vi "REST API Test.vi"() -> ()   [LabVIEW 2017]
uses:
  <vilib>/addons/_JKI.lib/REST Client/classes/REST Client/REST Client.lvclass
  Bridge Configuration.ctl
  Result Configuration.ctl
panel:
  out "Console":string
  in  "Exit":bool
  out "Vout, V":dbl=110.0 step=100.0
  in  "Post":bool
  in  "Get":bool
  in  "R4, Ohm":dbl min=0.0 step=100.0
  in  "R3, Ohm":dbl min=0.0 step=100.0
  in  "R2, Ohm":dbl min=0.0 step=100.0
  in  "R1, Ohm":dbl min=0.0 step=100.0
  in  "Vin, V":dbl step=100.0
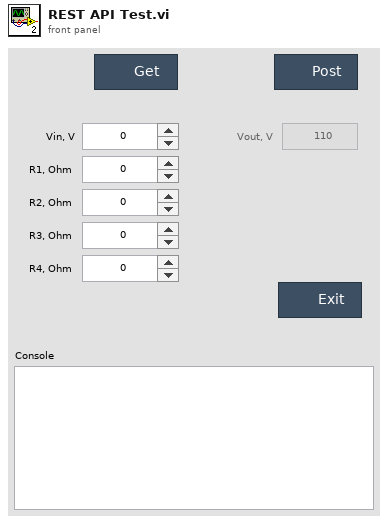
[diagram p1: front panel]
types:
  T1 = enum32{"Invalid", "Standard", "Closed", "Hidden", "Minimized", "Maximized"}
  T2 = enum32{"invalid app kind", "Development System", "Run Time System", "Student Edition", "Embedded LabVIEW", "Evaluation", "Custom"}
  T3 = typedef "Bridge Configuration.ctl" = cluster{"Vin":dbl, "R1":dbl, "R2":dbl, "R3":dbl, "R4":dbl}
  T4 = typedef "Result Configuration.ctl" = cluster{"Vout":dbl}
  T5 = cluster{"Core":cluster{"Current VI Reference":refnum<vi>, "Close Panel on Exit?":bool}, "REST Client":refnum<class "REST Client.lvclass">, "Bridge Configuration":T3, "Vout":dbl}
  T6 = cluster{"Current VI Reference":refnum<vi>, "Close Panel on Exit?":bool}
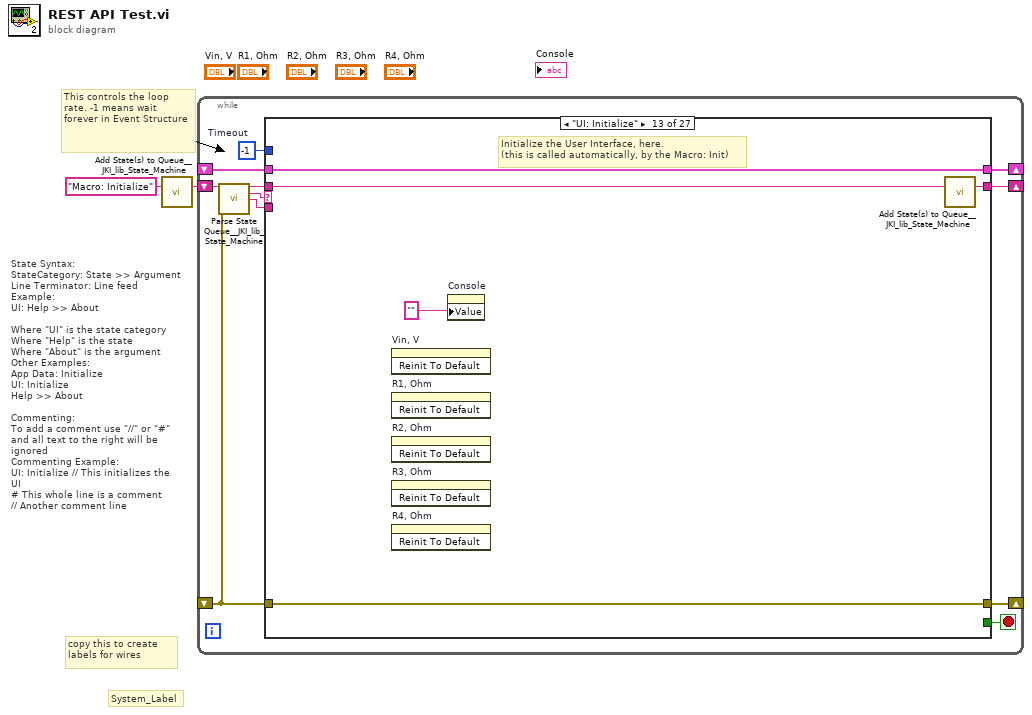
[diagram p0: block diagram]
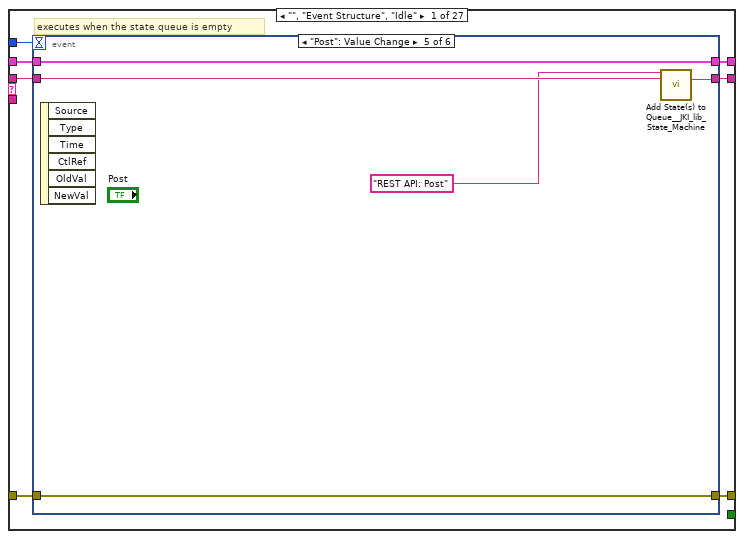
[diagram p2: hidden frame]
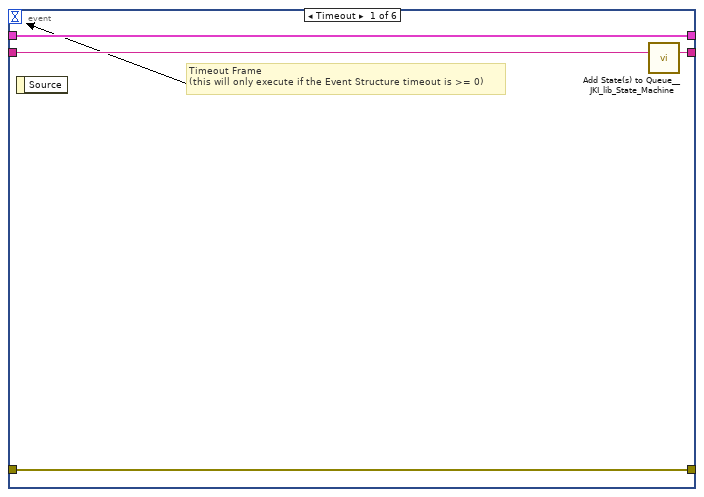
[diagram p3: hidden frame]
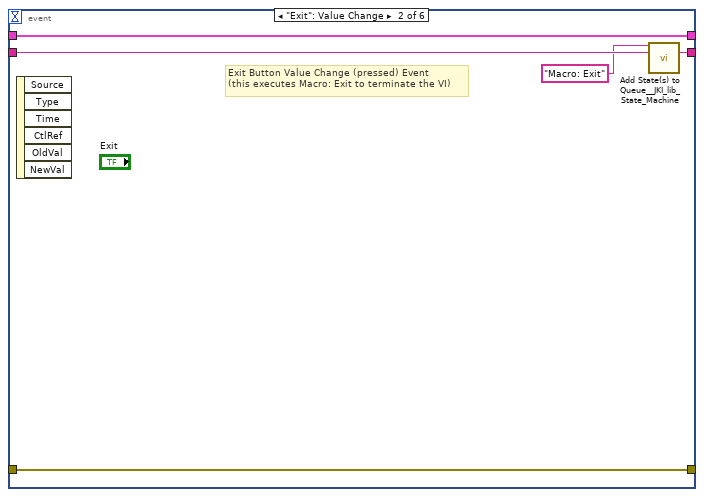
[diagram p4: hidden frame]
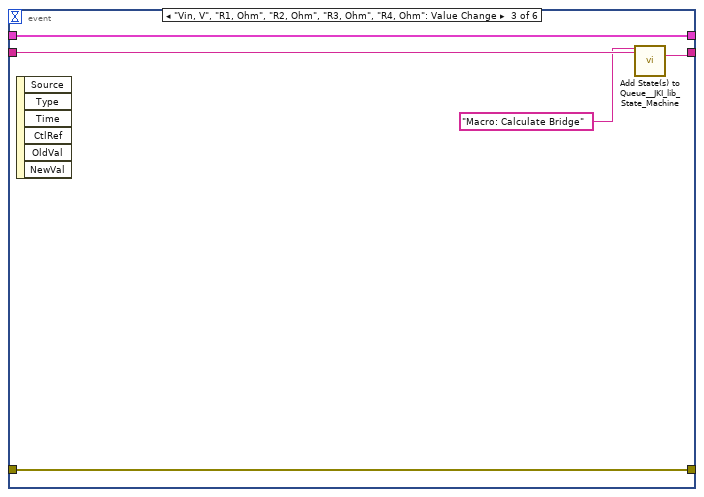
[diagram p5: hidden frame]
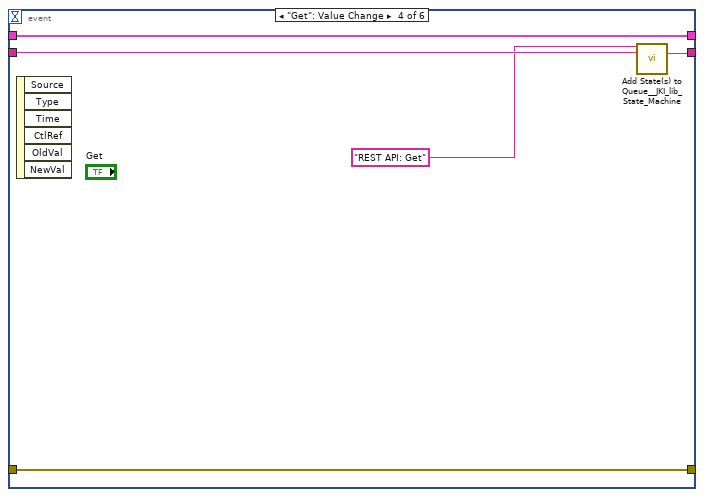
[diagram p6: hidden frame]
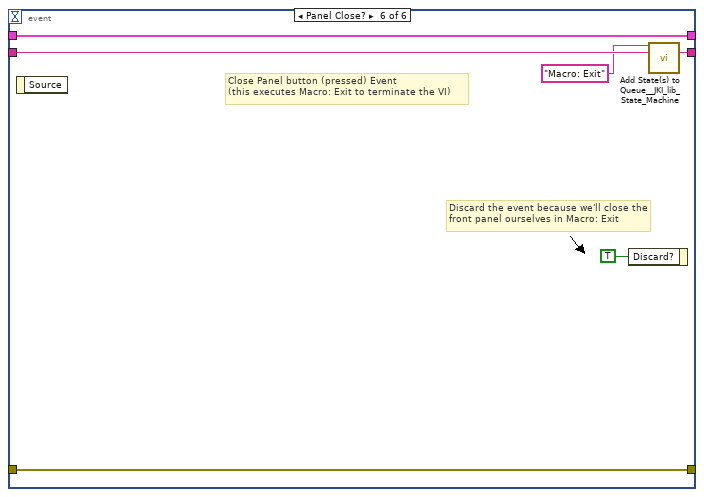
[diagram p7: hidden frame]
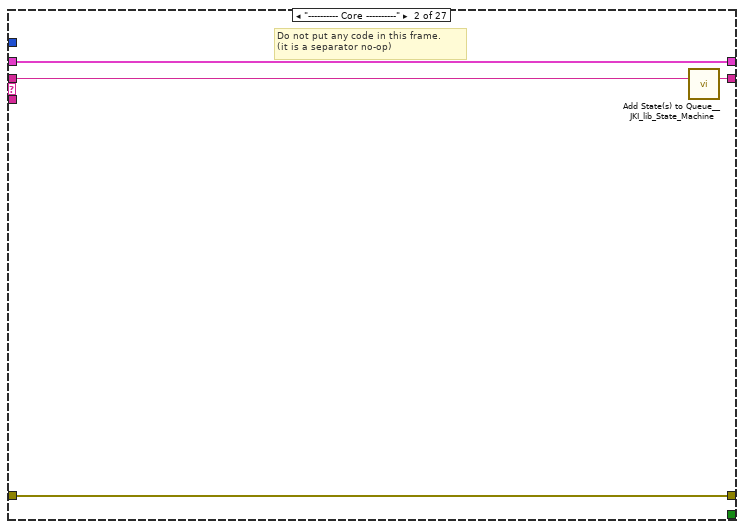
[diagram p8: hidden frame]
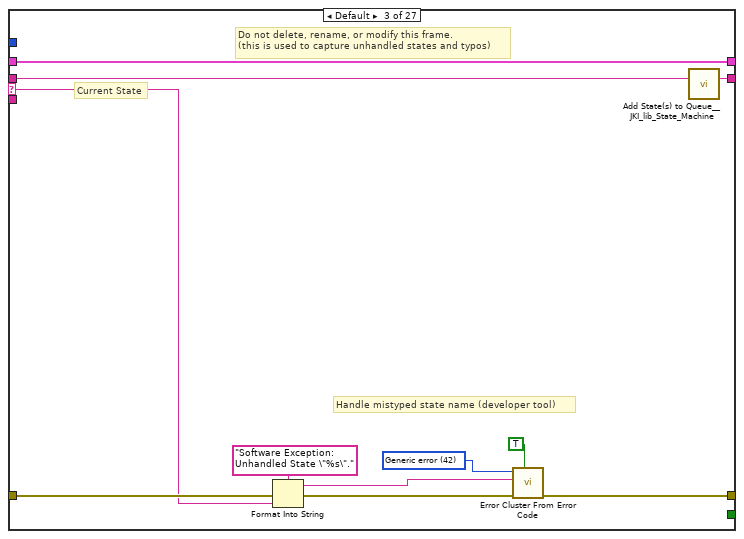
[diagram p9: hidden frame]
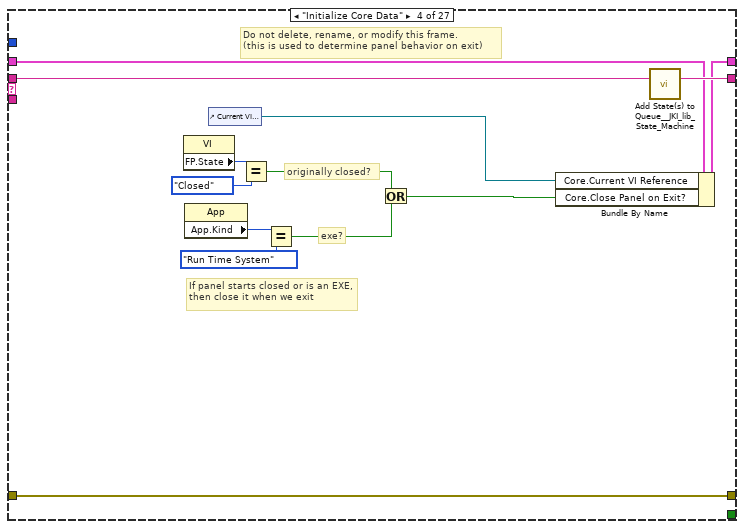
[diagram p10: hidden frame]
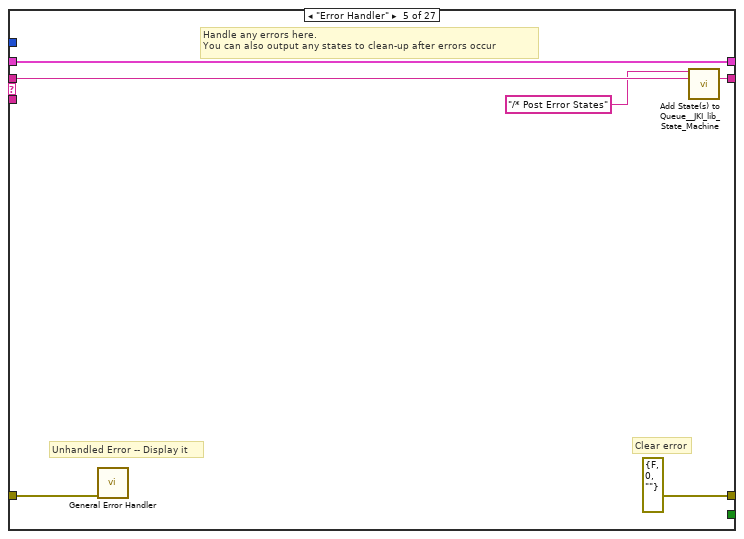
[diagram p11: hidden frame]
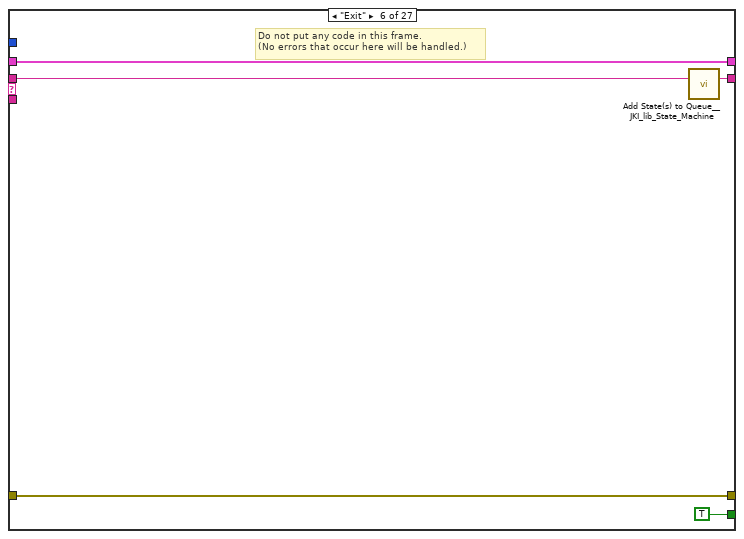
[diagram p12: hidden frame]
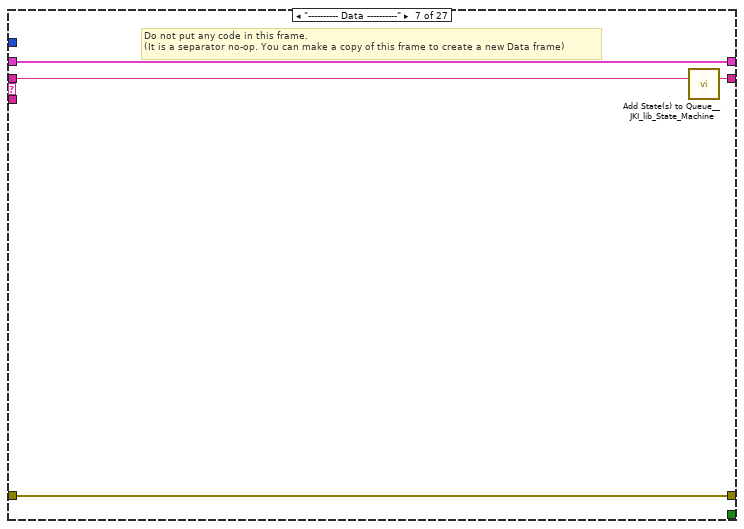
[diagram p13: hidden frame]
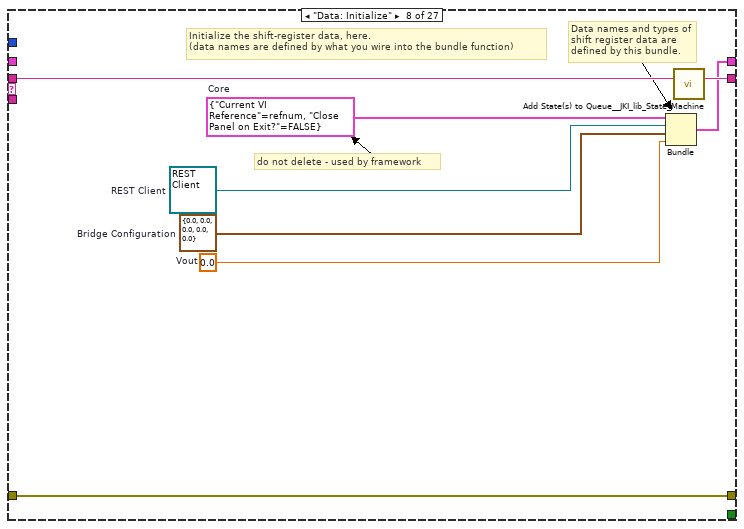
[diagram p14: hidden frame]
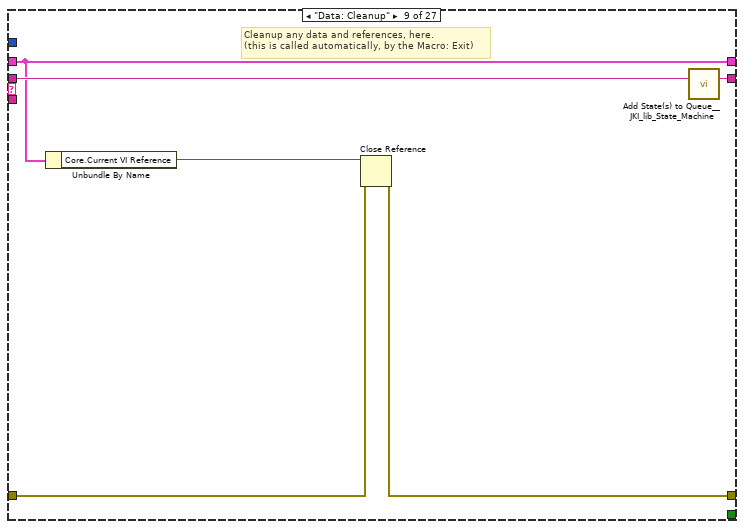
[diagram p15: hidden frame]
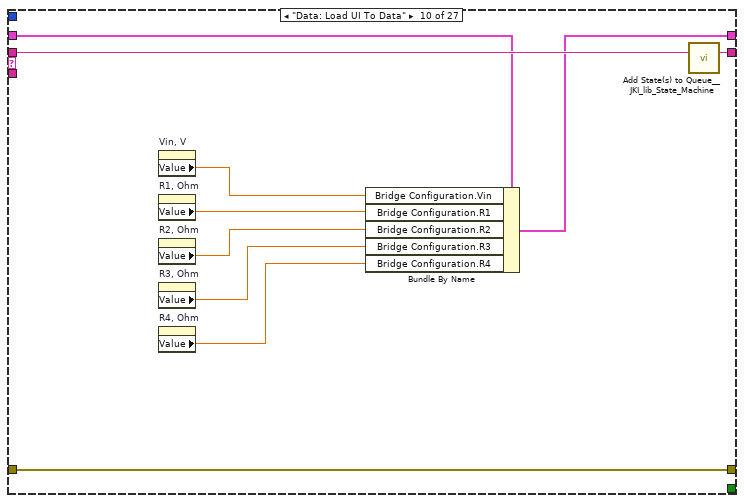
[diagram p16: hidden frame]
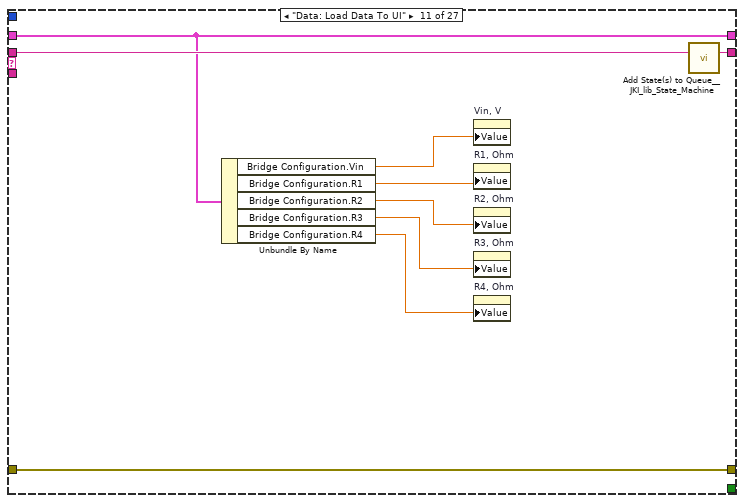
[diagram p17: hidden frame]
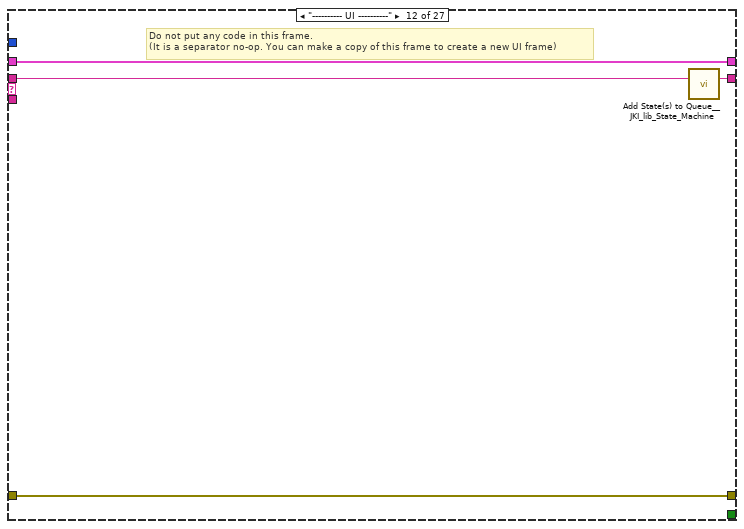
[diagram p18: hidden frame]
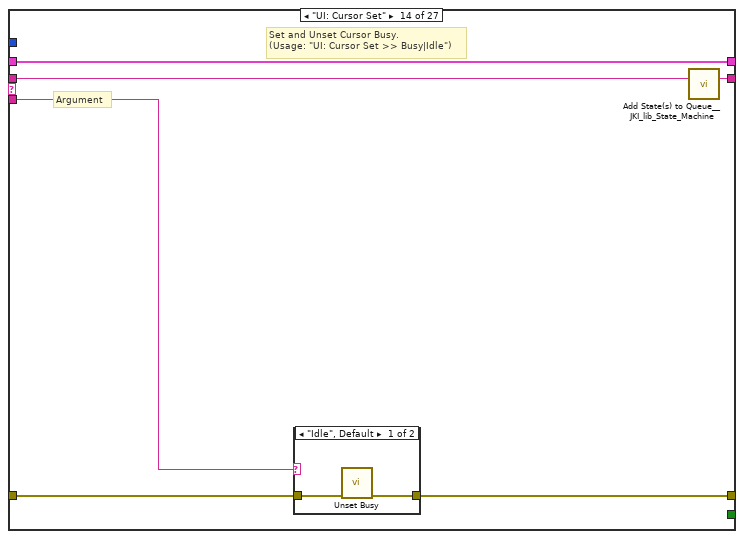
[diagram p19: hidden frame]
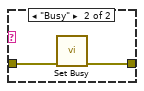
[diagram p20: hidden frame]
diagram:
  # "State Syntax:\nStateCategory: State >> Argument\nLine Terminator: Line feed\nExample:\nUI: Help >> About\n\nWhere \"UI\" is the state category\nWhere \"Help\" is the state\nWhere \"About\" is the argument\nOther Examples:\nApp Data: Initialize\nUI: Initialize\nHelp >> About\n\nCommenting:\nTo add a comment use \"//\" or \"#\" and all text to the right will be ignored\nCommenting Example:\nUI: Initialize // This initializes the UI\n# This whole line is a comment\n// Another comment line"
  # "copy this to create labels for wires"
  # "This controls the loop rate. -1 means wait forever in Event Structure"
  # "System_Label"
  n1 = call <vilib>:"Add State(s) to Queue__JKI_lib_State_Machine.vi"("State(s) in (\"\")"="Macro: Initialize") -> ("States Out"=w2:string)  [unwired: 14 in]
  n2 = while {
    shift-right: [w6] -> _
    shift-left: _ -> [w5]
    shift-right: [w9] -> _
    shift-left: _ -> [w3]
    shift-right: [w8] -> _
    shift-left: w2 -> [w10]
    stop <- w7 stop-if-true
    w4 = -1  # Timeout
    n3 = call <vilib>:"Parse State Queue__JKI_lib_State_Machine.vi"("State Queue"=w10, "Error In (no error)"=w3) -> ("Remaining States"=w12:string, "Current State"=w13:string, "Arguments"=w11:string)  [unwired: 11 in]
    n4 = case shown="\"UI: Initialize\"" w13 {
      selector: w13 -> [_ _ w55 _ _ _ _ _ _ _ _ _ _ _ _ _ _ _ _ _ _ _ _ _ _ _ _]
      tunnel: w12 -> [w20 w54 w59 w78 w84 w89 w93 w101 w107 w117 w126 w130 w135 w141 w152 w222 w226 w232 w237 w247 w251 w259 w272 w285 w291 w295 w306]
      tunnel: w11 -> [_ _ _ _ _ _ _ _ _ _ _ _ _ w136 w146 _ _ _ _ _ _ _ _ _ _ _ _]
      tunnel: w5 -> [w18 w51 w57 w71 w81 w87 w90 _ w102 w109 w118 w127 w133 w139 w148 w219 w223 w229 w234 w244 w248 w257 w264 w283 w289 w292 w298]
      tunnel: [w17 w52 w61 w75 errorcluster {"status"=FALSE, "code"=0, "source"=""} ("error out") w86 w91 w98 w103 w115 w124 w128 w132 w137 w149 w220 w224 w230 w235 w245 w249 w252 w265 w273 w286 w293 w304] -> w9
      tunnel: w3 -> [w16 w52 w60 w75 w80 w86 w91 w98 w104 w115 w124 w128 w132 w138 w150 w220 w224 w230 w235 w245 w249 w253 w267 w278 w287 w293 w304]
      tunnel: [w19 w53 w58 w77 w83 w88 w92 w100 w106 w116 w125 w129 w134 w140 w151 w221 w225 w231 w236 w246 w250 w258 w271 w284 w290 w294 w305] -> w8
      tunnel: [_ _ _ _ _ TRUE _ _ _ _ _ _ _ _ _ _ _ _ _ _ _ _ _ _ _ _ _] -> w7
      tunnel: [w15 w51 w57 w76 w81 w87 w90 w99 w102 w108 w118 w127 w133 w139 w148 w219 w223 w229 w234 w244 w248 w256 w262 w283 w289 w292 w296] -> w6
      tunnel: w4 -> [w14 _ _ _ _ _ _ _ _ _ _ _ _ _ _ _ _ _ _ _ _ _ _ _ _ _ _]
      frame "", "Event Structure", "Idle" {
        # "executes when the state queue is empty"
        n5 = event shown="[4] \"Post\": Value Change" {
          selector: _ -> [_ _ _ _ _ _]
          dyn-events: _ -> [_ _ _ _ _ _]
          timeout: w14 -> [_ _ _ _ _ _]
          tunnel: w20 -> [w24 w29 w33 w37 w42 w50]
          tunnel: [w23 w28 w34 w38 w43 w49] -> w19
          tunnel: w18 -> [w21 w26 w31 w39 w44 w47]
          tunnel: [w22 w27 w32 w36 w41 w48] -> w17
          tunnel: w16 -> [w22 w27 w32 w36 w41 w48]
          tunnel: [w21 w26 w31 w39 w44 w47] -> w15
          event Timeout {
            # "Timeout Frame\n(this will only execute if the Event Structure timeout is >= 0)"
            n6 = event-data() -> ()  [unwired: 1 in, 1 out]
            n7 = call <vilib>:"Add State(s) to Queue__JKI_lib_State_Machine.vi"("State(s) in (\"\")"=w24) -> ("States Out"=w23:string)  [unwired: 14 in]
          }
          event "Exit": Value Change {
            # "Exit Button Value Change (pressed) Event\n(this executes Macro: Exit to terminate the VI)"
            n8 = event-data() -> ()  [unwired: 1 in, 6 out]
            n9 = call <vilib>:"Add State(s) to Queue__JKI_lib_State_Machine.vi"("State(s) in Front (\"\")"="Macro: Exit", "State(s) in (\"\")"=w29) -> ("States Out"=w28:string)  [unwired: 13 in]
          }
          event "Vin, V", "R1, Ohm", "R2, Ohm", "R3, Ohm", "R4, Ohm": Value Change {
            n10 = event-data() -> ()  [unwired: 1 in, 6 out]
            n11 = call <vilib>:"Add State(s) to Queue__JKI_lib_State_Machine.vi"("State(s) in Front (\"\")"="Macro: Calculate Bridge", "State(s) in (\"\")"=w33) -> ("States Out"=w34:string)  [unwired: 13 in]
          }
          event "Get": Value Change {
            n12 = event-data() -> ()  [unwired: 1 in, 6 out]
            n13 = call <vilib>:"Add State(s) to Queue__JKI_lib_State_Machine.vi"("State(s) in Front (\"\")"="REST API: Get" ("State(s) in Front (\"\")"), "State(s) in (\"\")"=w37) -> ("States Out"=w38:string)  [unwired: 13 in]
          }
          event "Post": Value Change {
            n14 = event-data() -> ()  [unwired: 1 in, 6 out]
            n15 = call <vilib>:"Add State(s) to Queue__JKI_lib_State_Machine.vi"("State(s) in Front (\"\")"="REST API: Post" ("State(s) in Front (\"\")"), "State(s) in (\"\")"=w42) -> ("States Out"=w43:string)  [unwired: 13 in]
          }
          event Panel Close? {
            # "Discard the event because we'll close the front panel ourselves in Macro: Exit"
            # "Close Panel button (pressed) Event\n(this executes Macro: Exit to terminate the VI)"
            n16 = event-data() -> ()  [unwired: 1 in, 1 out]
            n17 = event-data("Discard?"=TRUE) -> ()  [unwired: 1 in, 1 out]
            n18 = call <vilib>:"Add State(s) to Queue__JKI_lib_State_Machine.vi"("State(s) in Front (\"\")"="Macro: Exit", "State(s) in (\"\")"=w50) -> ("States Out"=w49:string)  [unwired: 13 in]
          }
        }
      }
      frame "---------- Core ----------" {
        # "Do not put any code in this frame.\n(it is a separator no-op)"
        n19 = call <vilib>:"Add State(s) to Queue__JKI_lib_State_Machine.vi"("State(s) in (\"\")"=w54) -> ("States Out"=w53:string)  [unwired: 14 in]
      }
      frame Default {
        w64 = 42 items=["No error", "Argument error", "Memory is full", "Out of zone", "End of file", "File already open", "Generic file I/O error", "File not found", "File permission error", "Disk is full", "Duplicate path", "Too many files open", "System feature not enabled", "Resource file not found", "Cannot add resource", "Resource not found", "Image not found", "Image memory error", "Pen does not exist", "Config type invalid", "Config token not found", "Config parse error", "Config memory error", "Bad external code format", "Bad external code offset", "External code not present", "Null window", "Destroy window error", "Null menu", "Print aborted", "Bad print record", "Print driver error", "Windows error during printing", "Memory error during printing", "Print dialog error", "Generic print error", "Invalid device refnum", "Device not found", "Device parameter error", "Device unit error", "Cannot open device", "Device call aborted", "Generic error", "Cancelled by user", "Object ID too low", "Object ID too high", "Object not in heap", "Unknown heap", "Unknown object (invalid DefProc)", "Unknown object (DefProc not in table)", "Message out of range", "Invalid (null) method", "Unknown message", "Manager call not supported", "Bad address", "Network operation in progress", "Network operation timed out", "Connection is busy", "Network attribute not supported", "Network error", "Address in use", "System out of memory", "Connection aborted", "Connection refused", "Not connected", "Already connected", "Connection closed", "Initialization error (interapplication manager)", "Bad occurrence", "Wait on unbound occurrence handler", "Occurrence queue overflow", "Datalog type conflict", "Unused", "Unrecognized type (interapplication manager)", "Memory corrupt", "Failed to make temporary DLL", "Old CIN version", "Drag socket not found", "Failed to load drop-object", "Failed to register OLE object", "Failed to release OLE object", "Format specifier type mismatch", "Unknown format specifier", "Too few format specifiers", "Too many format specifiers", "Scan failed", "Newer CIN version", "Error converting to variant", "Runtime menu error", "Password tampered", "Variant attribute not found", "Incompatible variant data type", "Event data is not available", "Event Store is not present", "Occurrence is not found", "Event Queue is not created", "Event info is not available", "Refnum passed is NULL", "Error retrieving Class GUID", "Error retrieving CoClass GUID", "Error retrieving TypeLib GUID.", "Bad built application magic bytes.", "Specific driver is different from the specific driver associated with the Logical Name.", "There is no session opened to the class driver.", "Max Error", "MAX - Error with config objects", "MAX - Error loading configuration", "MAX - Group not supported"]
        # "Current State"
        # "Do not delete, rename, or modify this frame.\n(this is used to capture unhandled states and typos)"
        # "Handle mistyped state name (developer tool)"
        n20 = Format Into String(format string="Software Exception: Unhandled State \"%s\"." ("message"), error in=w60, w55) -> (resulting string=w63:string, error out=w62:errorcluster)  [unwired: 1 in]
        n21 = call <vilib>:"Error Cluster From Error Code.vi"("show call chain? (False)"=TRUE, "error in (no error)"=w62, "error message (\"\")"=w63, "error code (0)"=w64) -> ("error out"=w61:errorcluster)  [unwired: 5 in]
        n22 = call <vilib>:"Add State(s) to Queue__JKI_lib_State_Machine.vi"("State(s) in (\"\")"=w59) -> ("States Out"=w58:string)  [unwired: 14 in]
      }
      frame "Initialize Core Data" {
        # "Do not delete, rename, or modify this frame.\n(this is used to determine panel behavior on exit)"
        # "originally closed?"
        # "exe?"
        # "If panel starts closed or is an EXE, then close it when we exit"
        n23 = property class="VI"() -> ("FP.State"=w68:T1)  [unwired: 2 in, 2 out]
        n24 = property class="App"() -> ("App.Kind"=w74:T2)  [unwired: 2 in, 2 out]
        n25 = control-ref of="Current VI Reference"() -> (w69:refnum<vi>)
        n26 = Equal?(x=w68, y=T1."Closed" ("Front Panel Window:State")) -> (x = y?=w66:bool)
        n27 = Equal?(x=w74, y=T2."Run Time System" ("Application:Kind")) -> (x = y?=w72:bool)
        n28 = Or(x=w66, y=w72) -> (x .or. y?=w70:bool)
        n29 = Bundle By Name(cluster=w71, "Core.Current VI Reference"=w69, "Core.Close Panel on Exit?"=w70) -> (w76:T5)
        n30 = call <vilib>:"Add State(s) to Queue__JKI_lib_State_Machine.vi"("State(s) in (\"\")"=w78) -> ("States Out"=w77:string)  [unwired: 14 in]
      }
      frame "Error Handler" {
        # "Unhandled Error -- Display it"
        # "Handle any errors here.\nYou can also output any states to clean-up after errors occur"
        # "Clear error"
        n31 = call <vilib>:"General Error Handler.vi"("error in (no error)"=w80) -> ()  [unwired: 10 in, 5 out]
        n32 = call <vilib>:"Add State(s) to Queue__JKI_lib_State_Machine.vi"("State(s) in Front (\"\")"="/* Post Error States", "State(s) in (\"\")"=w84) -> ("States Out"=w83:string)  [unwired: 13 in]
      }
      frame "Exit" {
        # "Do not put any code in this frame.\n(No errors that occur here will be handled.)"
        n33 = call <vilib>:"Add State(s) to Queue__JKI_lib_State_Machine.vi"("State(s) in (\"\")"=w89) -> ("States Out"=w88:string)  [unwired: 14 in]
      }
      frame "---------- Data ----------" {
        # "Do not put any code in this frame.\n(It is a separator no-op. You can make a copy of this frame to create a new Data frame)"
        n34 = call <vilib>:"Add State(s) to Queue__JKI_lib_State_Machine.vi"("State(s) in (\"\")"=w93) -> ("States Out"=w92:string)  [unwired: 14 in]
      }
      frame "Data: Initialize" {
        w94 = 0.0  # Vout
        w95 = T3 {"Vin"=0.0, "R1"=0.0, "R2"=0.0, "R3"=0.0, "R4"=0.0}  # Bridge Configuration
        w96 = refnum<class "REST Client.lvclass"> refnum  # REST Client
        w97 = T6 {"Current VI Reference"=refnum, "Close Panel on Exit?"=FALSE}  # Core
        # "do not delete - used by framework"
        # "Data names and types of shift register data are defined by this bundle."
        # "Initialize the shift-register data, here.\n(data names are defined by what you wire into the bundle function)"
        n35 = Bundle("Core"=w97, "REST Client"=w96, "Bridge Configuration"=w95, "Vout"=w94) -> (w99:T5)  [unwired: 1 in]
        n36 = call <vilib>:"Add State(s) to Queue__JKI_lib_State_Machine.vi"("State(s) in (\"\")"=w101) -> ("States Out"=w100:string)  [unwired: 14 in]
      }
      frame "Data: Cleanup" {
        # "Cleanup any data and references, here.\n(this is called automatically, by the Macro: Exit)"
        n37 = Unbundle By Name(w102) -> ("Core.Current VI Reference"=w105:refnum<vi>)
        n38 = Close Reference(reference=w105, error in (no error)=w104) -> (error out=w103:errorcluster)
        n39 = call <vilib>:"Add State(s) to Queue__JKI_lib_State_Machine.vi"("State(s) in (\"\")"=w107) -> ("States Out"=w106:string)  [unwired: 14 in]
      }
      frame "Data: Load UI To Data" {
        n40 = property on="Vin, V" class="DigNum (strict)"() -> ("Value"=w114:dbl)  [unwired: 2 in, 2 out]
        n41 = property on="R1, Ohm" class="DigNum (strict)"() -> ("Value"=w113:dbl)  [unwired: 2 in, 2 out]
        n42 = property on="R2, Ohm" class="DigNum (strict)"() -> ("Value"=w112:dbl)  [unwired: 2 in, 2 out]
        n43 = property on="R3, Ohm" class="DigNum (strict)"() -> ("Value"=w111:dbl)  [unwired: 2 in, 2 out]
        n44 = property on="R4, Ohm" class="DigNum (strict)"() -> ("Value"=w110:dbl)  [unwired: 2 in, 2 out]
        n45 = Bundle By Name(cluster=w109, "Bridge Configuration.Vin"=w114, "Bridge Configuration.R1"=w113, "Bridge Configuration.R2"=w112, "Bridge Configuration.R3"=w111, "Bridge Configuration.R4"=w110) -> (w108:T5)
        n46 = call <vilib>:"Add State(s) to Queue__JKI_lib_State_Machine.vi"("State(s) in (\"\")"=w117) -> ("States Out"=w116:string)  [unwired: 14 in]
      }
      frame "Data: Load Data To UI" {
        n47 = Unbundle By Name(w118) -> ("Bridge Configuration.Vin"=w123:dbl, "Bridge Configuration.R1"=w122:dbl, "Bridge Configuration.R2"=w121:dbl, "Bridge Configuration.R3"=w120:dbl, "Bridge Configuration.R4"=w119:dbl)
        n48 = property on="Vin, V" class="DigNum (strict)"("Value"=w123) -> ()  [unwired: 2 in, 2 out]
        n49 = property on="R1, Ohm" class="DigNum (strict)"("Value"=w122) -> ()  [unwired: 2 in, 2 out]
        n50 = property on="R2, Ohm" class="DigNum (strict)"("Value"=w121) -> ()  [unwired: 2 in, 2 out]
        n51 = property on="R3, Ohm" class="DigNum (strict)"("Value"=w120) -> ()  [unwired: 2 in, 2 out]
        n52 = property on="R4, Ohm" class="DigNum (strict)"("Value"=w119) -> ()  [unwired: 2 in, 2 out]
        n53 = call <vilib>:"Add State(s) to Queue__JKI_lib_State_Machine.vi"("State(s) in (\"\")"=w126) -> ("States Out"=w125:string)  [unwired: 14 in]
      }
      frame "---------- UI ----------" {
        # "Do not put any code in this frame.\n(It is a separator no-op. You can make a copy of this frame to create a new UI frame)"
        n54 = call <vilib>:"Add State(s) to Queue__JKI_lib_State_Machine.vi"("State(s) in (\"\")"=w130) -> ("States Out"=w129:string)  [unwired: 14 in]
      }
      frame "UI: Initialize" {
        # "Initialize the User Interface, here.\n(this is called automatically, by the Macro: Init)"
        n55 = invoke on="Vin, V" class="DigNum (strict)" method="Reinit To Default"() -> ()  [unwired: 3 in, 3 out]
        n56 = invoke on="R1, Ohm" class="DigNum (strict)" method="Reinit To Default"() -> ()  [unwired: 3 in, 3 out]
        n57 = invoke on="R2, Ohm" class="DigNum (strict)" method="Reinit To Default"() -> ()  [unwired: 3 in, 3 out]
        n58 = invoke on="R3, Ohm" class="DigNum (strict)" method="Reinit To Default"() -> ()  [unwired: 3 in, 3 out]
        n59 = invoke on="R4, Ohm" class="DigNum (strict)" method="Reinit To Default"() -> ()  [unwired: 3 in, 3 out]
        n60 = property on="Console" class="Str"("Value"="" ("Console")) -> ()  [unwired: 2 in, 2 out]
        n61 = call <vilib>:"Add State(s) to Queue__JKI_lib_State_Machine.vi"("State(s) in (\"\")"=w135) -> ("States Out"=w134:string)  [unwired: 14 in]
      }
      frame "UI: Cursor Set" {
        # "Argument"
        # "Set and Unset Cursor Busy.\n(Usage: \"UI: Cursor Set >> Busy|Idle\")"
        n62 = case shown="\"Idle\", Default" w136 {
          tunnel: w138 -> [w143 w145]
          tunnel: [w142 w144] -> w137
          frame "Idle", Default {
            n63 = call <vilib>:"Unset Busy.vi"("error in (no error)"=w143) -> ("error out"=w142:errorcluster)  [unwired: 10 in]
          }
          frame "Busy" {
            n64 = call <vilib>:"Set Busy.vi"("error in (no error)"=w145) -> ("error out"=w144:errorcluster)  [unwired: 9 in, 1 out]
          }
        }
        n65 = call <vilib>:"Add State(s) to Queue__JKI_lib_State_Machine.vi"("State(s) in (\"\")"=w141) -> ("States Out"=w140:string)  [unwired: 14 in]
      }
      frame "UI: Front Panel State" {
        # "Argument"
        # "Set Front Panel Open or Closed\n(Usage: \"UI: Front Panel State >> Open|Close\")"
        n66 = Unbundle By Name(w148) -> ("Core.Current VI Reference"=w147:refnum<vi>)
        n67 = case shown="\"Minimize\", \"Minimized\"" w146 {
          tunnel: w150 -> [w158 w173 w184 w197 w210]
          tunnel: [w160 w174 w186 w199 w212] -> w149
          tunnel: w147 -> [w159 w171 w185 w198 w211]
          frame "Open", "Standard", Default {
            w153 = T1."Standard" ("State")
            n68 = property class="VI"(reference=w159, error in=w158) -> (reference out=w156:refnum<vi>, error out=w157:errorcluster, "FP.State"=w155:T1)
            n69 = Not Equal?(x=w155, y=w153) -> (x != y?=w154:bool)
            n70 = case shown="True" w154 {
              tunnel: [w164 w166] -> w160
              tunnel: w157 -> [w163 w166]
              tunnel: w156 -> [w162 _]
              tunnel: w153 -> [w161 _]
              frame True {
                n71 = invoke class="VI" method="FP.Open"(reference=w162, error in=w163, "Activate"=TRUE, "State"=w161) -> (error out=w164:errorcluster)  [unwired: 1 in, 4 out]
              }
              frame False {
              }
            }
          }
          frame "Close", "Closed" {
            n72 = property class="VI"(reference=w171, error in=w173) -> (reference out=w170:refnum<vi>, error out=w172:errorcluster, "FP.State"=w168:T1)
            n73 = Not Equal?(x=w168, y=T1."Closed" ("Front Panel Window:State")) -> (x != y?=w167:bool)
            n74 = case shown="True" w167 {
              tunnel: [w175 w178] -> w174
              tunnel: w172 -> [w175 w177]
              tunnel: w170 -> [_ w176]
              frame False {
              }
              frame True {
                n75 = invoke class="VI" method="FP.Close"(reference=w176, error in=w177) -> (error out=w178:errorcluster)  [unwired: 1 in, 2 out]
              }
            }
          }
          frame "Hidden", "Hide" {
            w179 = T1."Hidden" ("State")
            n76 = property class="VI"(reference=w185, error in=w184) -> (reference out=w182:refnum<vi>, error out=w183:errorcluster, "FP.State"=w181:T1)
            n77 = Not Equal?(x=w181, y=w179) -> (x != y?=w180:bool)
            n78 = case shown="True" w180 {
              tunnel: [w190 w191] -> w186
              tunnel: w183 -> [w189 w191]
              tunnel: w182 -> [w188 _]
              tunnel: w179 -> [w187 _]
              frame True {
                n79 = invoke class="VI" method="FP.Open"(reference=w188, error in=w189, "State"=w187) -> (error out=w190:errorcluster)  [unwired: 2 in, 4 out]
              }
              frame False {
              }
            }
          }
          frame "Minimize", "Minimized" {
            w192 = T1."Minimized" ("State")
            n80 = property class="VI"(reference=w198, error in=w197) -> (reference out=w195:refnum<vi>, error out=w196:errorcluster, "FP.State"=w194:T1)
            n81 = Not Equal?(x=w194, y=w192) -> (x != y?=w193:bool)
            n82 = case shown="True" w193 {
              tunnel: [w203 w204] -> w199
              tunnel: w196 -> [w202 w204]
              tunnel: w195 -> [w201 _]
              tunnel: w192 -> [w200 _]
              frame True {
                n83 = invoke class="VI" method="FP.Open"(reference=w201, error in=w202, "State"=w200) -> (error out=w203:errorcluster)  [unwired: 2 in, 4 out]
              }
              frame False {
              }
            }
          }
          frame "Maximize", "Maximized" {
            w205 = T1."Maximized" ("State")
            n84 = property class="VI"(reference=w211, error in=w210) -> (reference out=w208:refnum<vi>, error out=w209:errorcluster, "FP.State"=w207:T1)
            n85 = Not Equal?(x=w207, y=w205) -> (x != y?=w206:bool)
            n86 = case shown="True" w206 {
              tunnel: [w216 w217] -> w212
              tunnel: w209 -> [w215 w217]
              tunnel: w208 -> [w214 _]
              tunnel: w205 -> [w213 _]
              frame True {
                n87 = invoke class="VI" method="FP.Open"(reference=w214, error in=w215, "State"=w213) -> (error out=w216:errorcluster)  [unwired: 2 in, 4 out]
              }
              frame False {
              }
            }
          }
        }
        n88 = call <vilib>:"Add State(s) to Queue__JKI_lib_State_Machine.vi"("State(s) in (\"\")"=w152) -> ("States Out"=w151:string)  [unwired: 14 in]
      }
      frame "UI: Update Vout" {
        n89 = Unbundle By Name(w219) -> ("Vout"=→"Vout, V":dbl)
        n90 = call <vilib>:"Add State(s) to Queue__JKI_lib_State_Machine.vi"("State(s) in (\"\")"=w222) -> ("States Out"=w221:string)  [unwired: 14 in]
      }
      frame "---------- Macro ----------" {
        # "Do not put any code in this frame.\n(It is a separator no-op. You can make a copy of this frame to create a new Macro frame)"
        n91 = call <vilib>:"Add State(s) to Queue__JKI_lib_State_Machine.vi"("State(s) in (\"\")"=w226) -> ("States Out"=w225:string)  [unwired: 14 in]
      }
      frame "Macro: Initialize" {
        w228 = "Data: Initialize\nInitialize Core Data\nREST API: Create\nUI: Initialize\nUI: Front Panel State >> Open"  # Data: Initialize Initialize Core Data REST API: Create UI: Initialize UI: Front Panel State >> Open
        # "Initialization Macro\n(This is called once, when the VI starts)"
        n92 = call <vilib>:"Add State(s) to Queue__JKI_lib_State_Machine.vi"("State(s) in Front (\"\")"=w228, "State(s) in (\"\")"=w232, "State(s) at Back (\"\")"="Macro: Calculate Bridge" ("State(s) in Front (\"\")")) -> ("States Out"=w231:string)  [unwired: 12 in]
      }
      frame "Macro: Calculate Bridge" {
        n93 = call <vilib>:"Add State(s) to Queue__JKI_lib_State_Machine.vi"("State(s) in Front (\"\")"="Data: Load UI To Data\nCalculation: Vout\nUI: Update Vout" ("State(s) in Front (\"\")"), "State(s) in (\"\")"=w237) -> ("States Out"=w236:string)  [unwired: 13 in]
      }
      frame "Macro: Exit" {
        # "Exit Macro\n(This is called once, when the VI exits)"
        n94 = Unbundle By Name(w244) -> ("Core.Close Panel on Exit?"=w243:bool)
        n95 = Select(t="UI: Front Panel State >> Close", s=w243, f="") -> (s? t:f=w240:string)
        n96 = call <vilib>:"Add State(s) to Queue__JKI_lib_State_Machine.vi"("State(s) in (\"\")"=w240, "State(s) at Back (\"\")"="REST API: Destroy\nData: Cleanup\nExit") -> ("States Out"=w238:string)  [unwired: 13 in]
        n97 = call <vilib>:"Add State(s) to Queue__JKI_lib_State_Machine.vi"("State(s) in Front (\"\")"=w238, "State(s) in (\"\")"=w247) -> ("States Out"=w246:string)  [unwired: 13 in]
      }
      frame "---------- REST API ----------" {
        # "Template Separator\n(You can make a copy of, or modify, this frame)"
        n98 = call <vilib>:"Add State(s) to Queue__JKI_lib_State_Machine.vi"("State(s) in (\"\")"=w251) -> ("States Out"=w250:string)  [unwired: 14 in]
      }
      frame "REST API: Create" {
        n99 = call <vilib>:"Create REST Client.vi"("error in (no error)"=w253, "Base URL"="http://localhost:3000") -> ("error out"=w252:errorcluster, "REST Client out"=w254:refnum<class "REST Client.lvclass">)  [unwired: 8 in]
        n100 = Bundle By Name(cluster=w257, "REST Client"=w254) -> (w256:T5)
        n101 = call <vilib>:"Add State(s) to Queue__JKI_lib_State_Machine.vi"("State(s) in (\"\")"=w259) -> ("States Out"=w258:string)  [unwired: 14 in]
      }
      frame "REST API: Get" {
        n102 = Unbundle By Name(w264) -> ("REST Client"=w270:refnum<class "REST Client.lvclass">)
        n103 = call-dynamic "HTTP GET.vi"("error in (no error)"=w267, "Path"="/bridge", "REST Client in"=w270) -> ("error out"=w266:errorcluster, "Response body"=w260:string)  [unwired: 3 in, 4 out]
        n104 = Unflatten From JSON(JSON string=w260, type and defaults=T3 {"Vin"=0.0, "R1"=0.0, "R2"=0.0, "R3"=0.0, "R4"=0.0} ("Bridge Configuration"), error in (no error)=w266) -> (value=w263:T3, error out=w265:errorcluster)  [unwired: 4 in]
        n105 = property on="Console" class="Str"("Value"=w260) -> ()  [unwired: 2 in, 2 out]
        n106 = Bundle By Name(cluster=w264, "Bridge Configuration"=w263) -> (w262:T5)
        n107 = call <vilib>:"Add State(s) to Queue__JKI_lib_State_Machine.vi"("State(s) in Front (\"\")"="Data: Load Data To UI\nMacro: Calculate Bridge" ("State(s) in Front (\"\")"), "State(s) in (\"\")"=w272) -> ("States Out"=w271:string)  [unwired: 13 in]
      }
      frame "REST API: Post" {
        n108 = property on="Vout, V" class="DigNum (strict)"() -> ("Value"=w280:dbl)  [unwired: 2 in, 2 out]
        n109 = Unbundle By Name(w283) -> ("REST Client"=w282:refnum<class "REST Client.lvclass">)
        n110 = Bundle By Name(cluster=T4 {"Vout"=0.0} ("Result"), "Vout"=w280) -> (w279:T4)
        n111 = Flatten To JSON(anything=w279, error in (no error)=w278) -> (JSON string=w276:string, 11:w277:errorcluster)  [unwired: 1 in]
        n112 = call-dynamic "HTTP POST.vi"("error in (no error)"=w277, "Request body"=w276, "Path"="/results", "REST Client in"=w282) -> ("error out"=w273:errorcluster, "Response body"=w274:string)  [unwired: 2 in, 4 out]
        n113 = property on="Console" class="Str"("Value"=w274) -> ()  [unwired: 2 in, 2 out]
        n114 = call <vilib>:"Add State(s) to Queue__JKI_lib_State_Machine.vi"("State(s) in (\"\")"=w285) -> ("States Out"=w284:string)  [unwired: 14 in]
      }
      frame "REST API: Destroy" {
        n115 = Unbundle By Name(w289) -> ("REST Client"=w288:refnum<class "REST Client.lvclass">)
        n116 = call-dynamic "Destroy REST Client.vi"("error in (no error)"=w287, "REST Client in"=w288) -> ("error out"=w286:errorcluster)  [unwired: 9 in]
        n117 = call <vilib>:"Add State(s) to Queue__JKI_lib_State_Machine.vi"("State(s) in (\"\")"=w291) -> ("States Out"=w290:string)  [unwired: 14 in]
      }
      frame "---------- Calculation ----------" {
        # "Template Separator\n(You can make a copy of, or modify, this frame)"
        n118 = call <vilib>:"Add State(s) to Queue__JKI_lib_State_Machine.vi"("State(s) in (\"\")"=w295) -> ("States Out"=w294:string)  [unwired: 14 in]
      }
      frame "Calculation: Vout" {
        n119 = Unbundle By Name(w298) -> ("Bridge Configuration.Vin"=w303:dbl, "Bridge Configuration.R1"=w302:dbl, "Bridge Configuration.R2"=w301:dbl, "Bridge Configuration.R3"=w300:dbl, "Bridge Configuration.R4"=w299:dbl)
        n120 = formula code="Vout=Vin*(R4/(R3+R4)-R2/(R1+R2));"("Vin"=w303, "R1"=w302, "R2"=w301, "R3"=w300, "R4"=w299) -> ("Vout"=w297:dbl)
        n121 = Bundle By Name(cluster=w298, "Vout"=w297) -> (w296:T5)
        n122 = call <vilib>:"Add State(s) to Queue__JKI_lib_State_Machine.vi"("State(s) in (\"\")"=w306) -> ("States Out"=w305:string)  [unwired: 14 in]
      }
    }
  }
